vi "Enqueue Time.vi"(10 "input cluster":T1, 11 "Time Interval (s)":dbl) -> ()   [LabVIEW 2019]
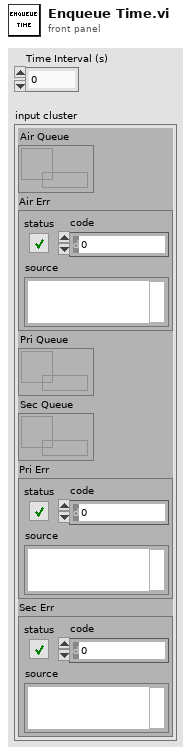
[diagram p1: front panel]
types:
  T1 = cluster{"Air Queue":refnum<queue>, "Air Err":errorcluster, "Pri Queue":refnum<queue>, "Sec Queue":refnum<queue>, "Pri Err":errorcluster, "Sec Err":errorcluster}
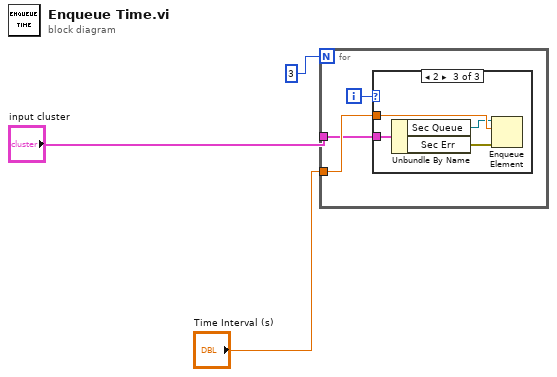
[diagram p0: block diagram]
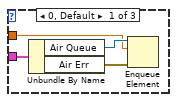
[diagram p2: hidden frame]
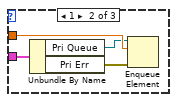
[diagram p3: hidden frame]
diagram:
  n1 = for {
    N: 3 -> [_]
    tunnel: "Time Interval (s)" -> [w6]
    tunnel: "input cluster" -> [w5]
    i -> [w4]
    n2 = case shown="2" w4 {
      tunnel: w6 -> [w7 w14 w18]
      tunnel: w5 -> [w8 w13 w17]
      frame 0, Default {
        n3 = Unbundle By Name(w8) -> ("Air Queue"=w10:refnum<queue>, "Air Err"=w9:errorcluster)
        n4 = Enqueue Element(queue=w10, element=w7, error in (no error)=w9) -> ()  [unwired: 1 in, 3 out]
      }
      frame 1 {
        n5 = Unbundle By Name(w13) -> ("Pri Queue"=w12:refnum<queue>, "Pri Err"=w11:errorcluster)
        n6 = Enqueue Element(queue=w12, element=w14, error in (no error)=w11) -> ()  [unwired: 1 in, 3 out]
      }
      frame 2 {
        n7 = Unbundle By Name(w17) -> ("Sec Queue"=w16:refnum<queue>, "Sec Err"=w15:errorcluster)
        n8 = Enqueue Element(queue=w16, element=w18, error in (no error)=w15) -> ()  [unwired: 1 in, 3 out]
      }
    }
  }
